vi "Set Build Specification Description.vi"(8 "error in (no error)":errorcluster, 10 "Build Specification Description":string, 11 "NI_AB_API_SDIST in":refnum<class "NI_AB_API_SDIST.lvclass">) -> (0 "error out":errorcluster, 3 "NI_AB_API_SDIST out":refnum<class "NI_AB_API_SDIST.lvclass">)   [LabVIEW 2020, in "NI_AB_API_SDIST.lvclass"]
uses:
  <vilib>/AppBuilder/AB_API/SDIST/NI_AB_API_SDIST.lvclass
  <vilib>/AppBuilder/AB_API/SDIST/NI_AB_API_SDIST.lvclass/NI_AB_API_SDIST.ctl
  <vilib>/AppBuilder/AB_API/Build/NI_AB_API_Build.lvclass
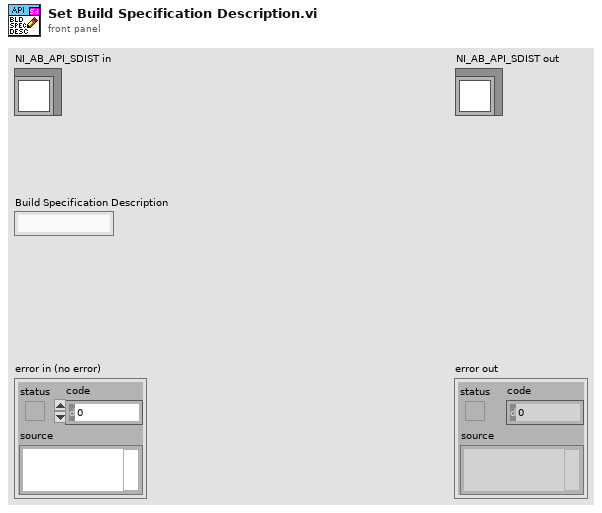
[diagram p1: front panel]
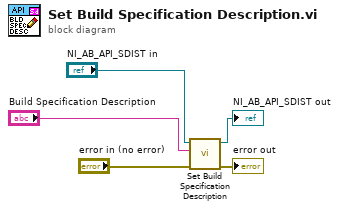
[diagram p0: block diagram]
diagram:
  n1 = call-parent "Set Build Specification Description.vi"("error in (no error)"="error in (no error)", "Build Specification Description"="Build Specification Description", "NI_AB_API_Build in"="NI_AB_API_SDIST in") -> ("error out"=→"error out":errorcluster, "NI_AB_API_Build out"=→"NI_AB_API_SDIST out":refnum<class "NI_AB_API_SDIST.lvclass">)  [unwired: 7 in]
